vi "pmu_Check Digital Names.vi"(8 "error in (no error)":errorcluster, 11 "digital names in":string[](array[string])) -> (0 "error out":errorcluster, 3 "digital names out":string[](array[string]))   [LabVIEW 2011, in "NI_EP_PMU.lvlib"]
uses:
  <vilib>/addons/Electrical Power/PMU/NI_EP_PMU.lvlib
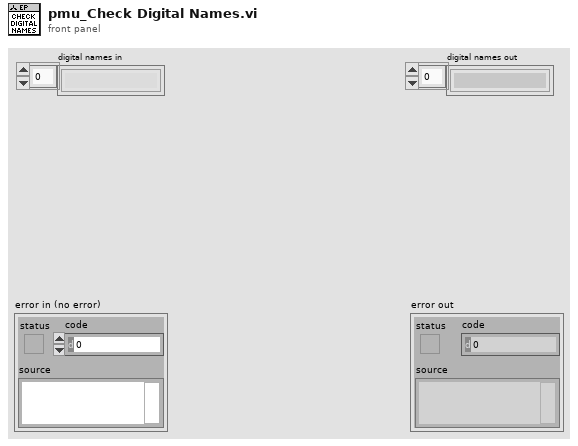
[diagram p1: front panel]
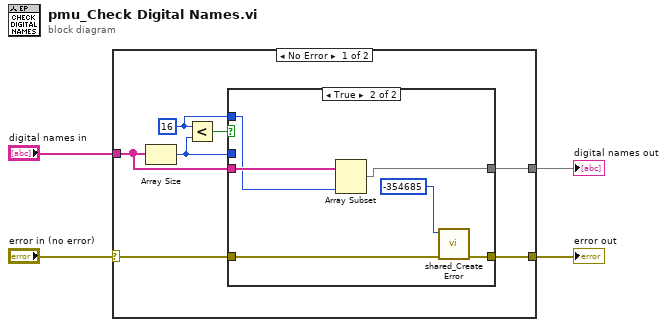
[diagram p0: block diagram]
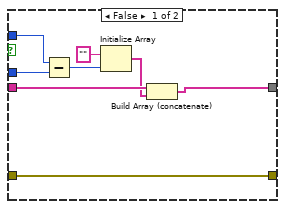
[diagram p2: hidden frame]
diagram:
  n1 = case shown="No Error" "error in (no error)" {
    selector: "error in (no error)" -> [w10 w26]
    tunnel: [w9 w26] -> w3
    tunnel: "digital names in" -> [w6 _]
    tunnel: [w5 _] -> w1
    frame No Error {
      w7 = 16 ("y")
      n2 = Array Size(array=w6) -> (size(s)=w8:i32)
      n3 = Less?(x=w7, y=w8) -> (x < y?=w11:bool)
      n4 = case shown="True" w11 {
        tunnel: w10 -> [w19 w21]
        tunnel: [w19 w20] -> w9
        tunnel: w8 -> [w17 _]
        tunnel: w7 -> [w18 w24]
        tunnel: w6 -> [w14 w25]
        tunnel: [w12 w23] -> w5
        frame False {
          n5 = Subtract(x=w18, y=w17) -> (x-y=w16:i32)
          n6 = Initialize Array("", w16) -> (w13:string[])
          n7 = Build Array (concatenate)(w14, w13) -> (w12:string[])
        }
        frame True {
          n8 = Array Subset(array=w25, length=w24) -> (w23:string[])  [unwired: 1 in]
          n9 = call <vilib>:"shared_Create Error.vi"("error in (no error)"=w21, "error code (0)"=-354685) -> ("error out"=w20:errorcluster)  [unwired: 9 in]
        }
      }
    }
    frame Error {
    }
  }
  "error out" <- w3
  "digital names out" <- w1
